vi "19052 PreSet_GR_CONT. _test.vi"(8 "error in (no error)":errorcluster, 10 "Step Time":dbl=0.001 min=0.0 max=99.9 step=0.1 format="%.1f", 11 "VISA resource in":refnum<visa-resource-name>) -> (0 "error out":errorcluster, 2 "output command":string, 3 "VISA resource out":refnum<visa-resource-name>)   [LabVIEW 2015]
doc: "This VI writes to the instrument the AC-V FREQ. value."
panel:
  # "Preset GR CONT."
  # "0=OFF\n0.1=KEY\n0.2-99.9 time to START"
  # "[sec]"
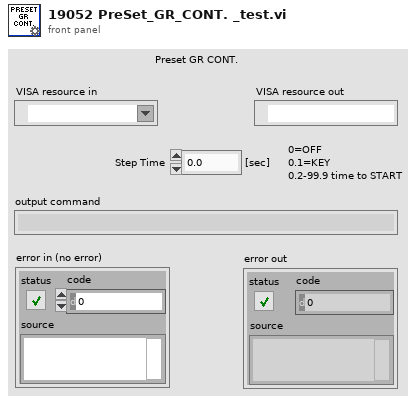
[diagram p1: front panel]
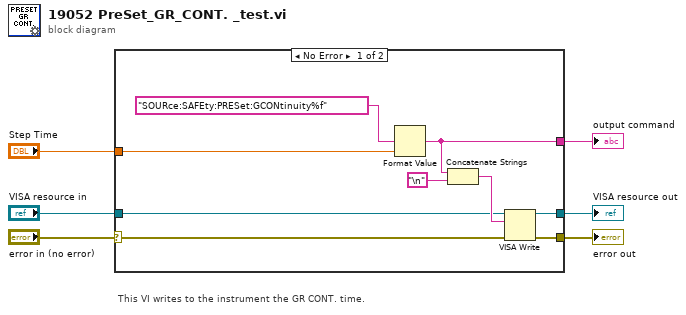
[diagram p0: block diagram]
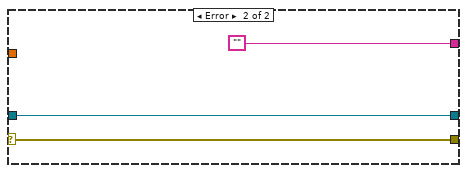
[diagram p2: hidden frame]
diagram:
  # "This VI writes to the instrument the GR CONT. time."
  n1 = case shown="No Error" "error in (no error)" {
    selector: "error in (no error)" -> [w14 w18]
    tunnel: [w15 w18] -> w6
    tunnel: "Step Time" -> [w10 _]
    tunnel: "VISA resource in" -> [w9 w17]
    tunnel: [w8 ""] -> w2
    tunnel: [w7 w17] -> w1
    frame No Error {
      n2 = Format Value(format string="SOURce:SAFEty:PRESet:GCONtinuity%f", value (0)=w10) -> (output string=w8:string)  [unwired: 1 in]
      n3 = Concatenate Strings(w8, "\n") -> (w11:string)
      n4 = VISA Write(VISA resource name=w9, write buffer=w11, error in (no error)=w14) -> (VISA resource name out=w7:refnum<visa-resource-name>, error out=w15:errorcluster)  [unwired: 1 out]
    }
    frame Error {
    }
  }
  "error out" <- w6
  "VISA resource out" <- w1
  "output command" <- w2
